vi "FGV_SQL_pinion_ID_buffer.vi"(4 "SQL_result":variant[][](array[variant]), 6 "connection reference":T2, 7 "options":T3, 8 "error_in":errorcluster, 9 "station":T1, 10 "PINION_ID":string, 11 "PINION_SERIAL":string) -> (0 "error_out":errorcluster, 2 "Pinion exists?":bool, 3 "ID_out":string)   [LabVIEW 2020]
uses:
  FGV_SQL_pinion_ID_buffer.ctl
  <vilib>/addons/database/Connection.llb/Conn ObjectReference.ctl
  STATION/station.ctl
  SQL_pinion_ID_buffer_all_info.ctl
  <vilib>/addons/database/NI_Database_API.lvlib
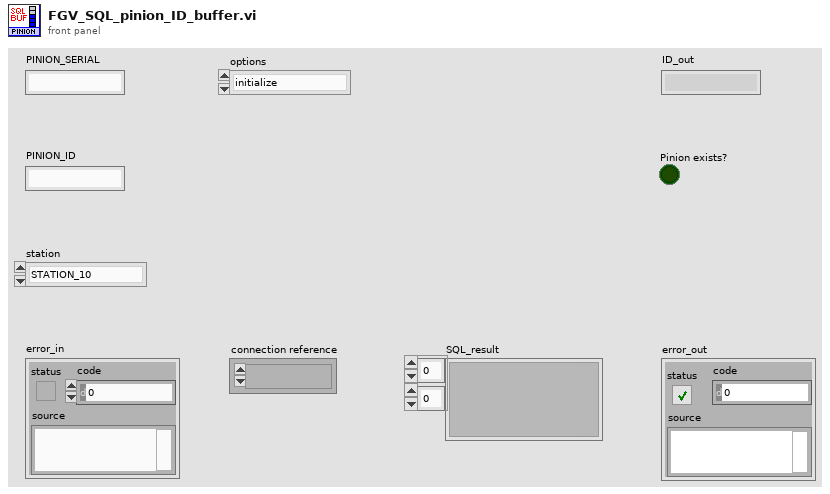
[diagram p1: front panel]
types:
  T1 = typedef "station.ctl" = enum16{"STATION_10", "STATION_20", "STATION_30", "STATION_40", "STATION_50", "STATION_60", "STATION_70", "STATION_80", "STATION_90", "STATION_100", "STATION_110", "STATION_120", "STATION_165", "MAIN"}
  T2 = typedef "NI_Database_API.lvlib/Conn ObjectReference.ctl" = refnum<k1>
  T3 = typedef "FGV_SQL_pinion_ID_buffer.ctl" = enum16{"initialize", "buffer_pinion_ID", "buffer_pinion_ID_SQL", "get_ID_for_name"}
  T4 = typedef "SQL_pinion_ID_buffer_all_info.ctl" = cluster{"PINION_SERIAL_and_ID":string[][], "PINION_SERIAL_and_ID_buffer_pos":i32, "PINION_SERIAL_and_ID_buffer_max_size":i32}
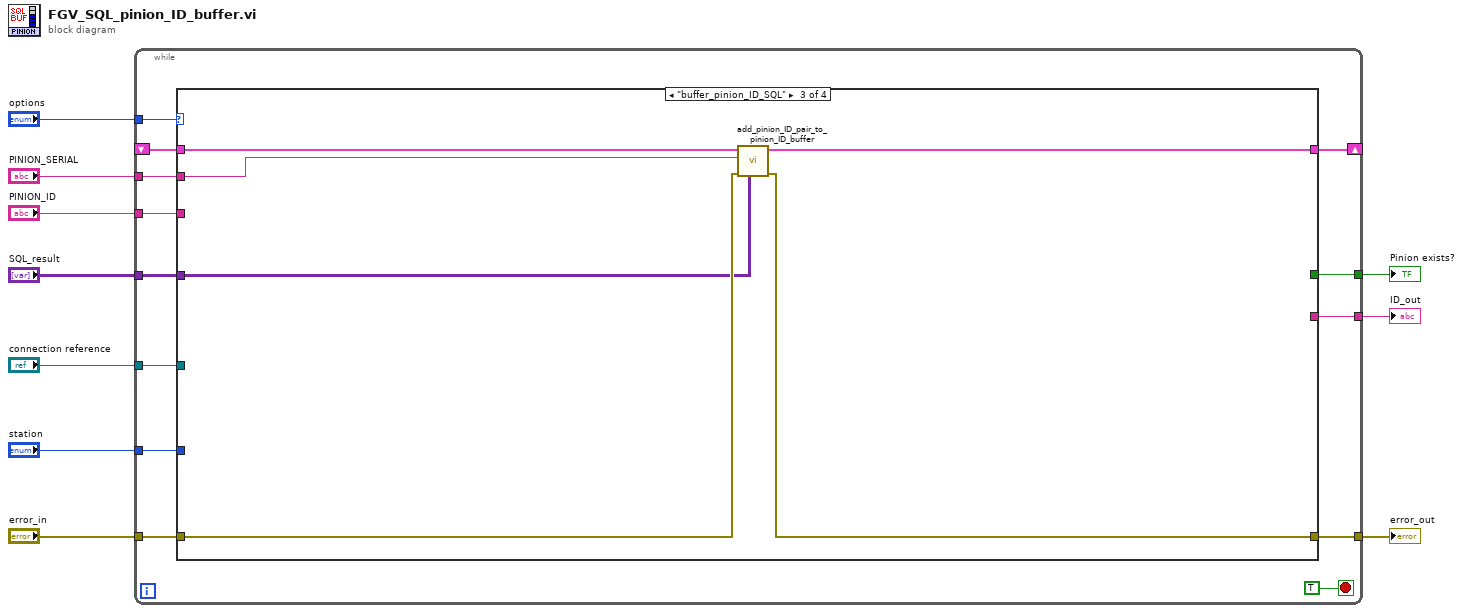
[diagram p0: block diagram]
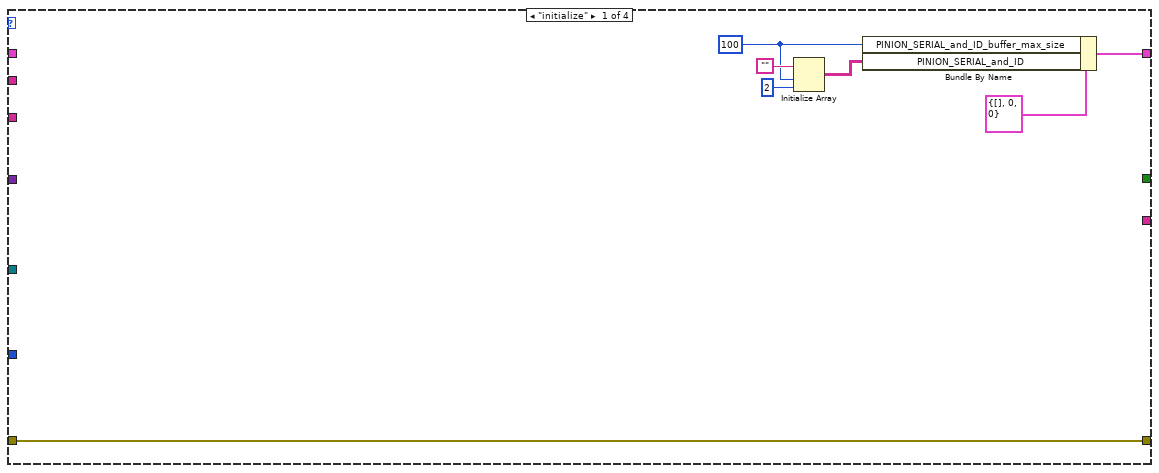
[diagram p2: hidden frame]
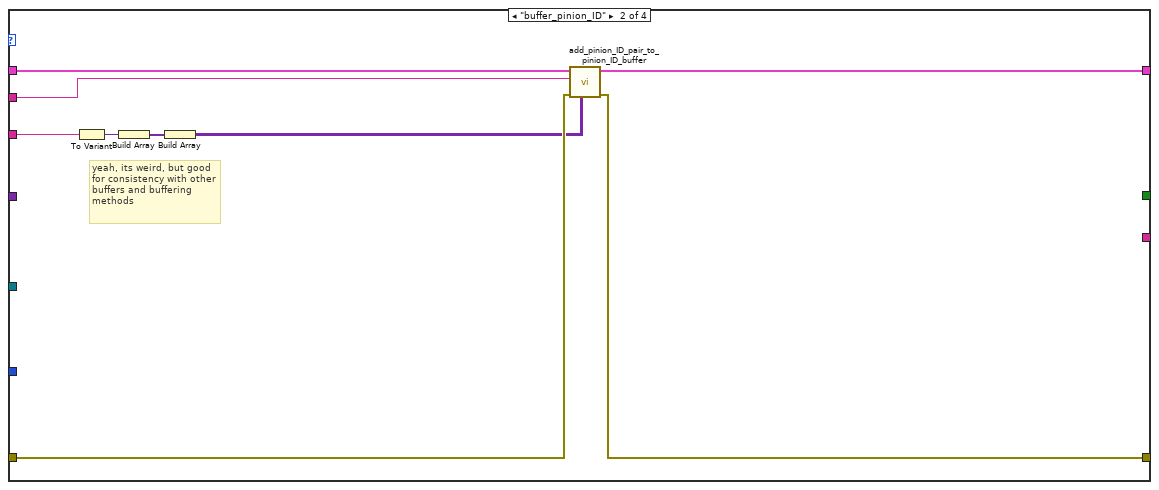
[diagram p3: hidden frame]
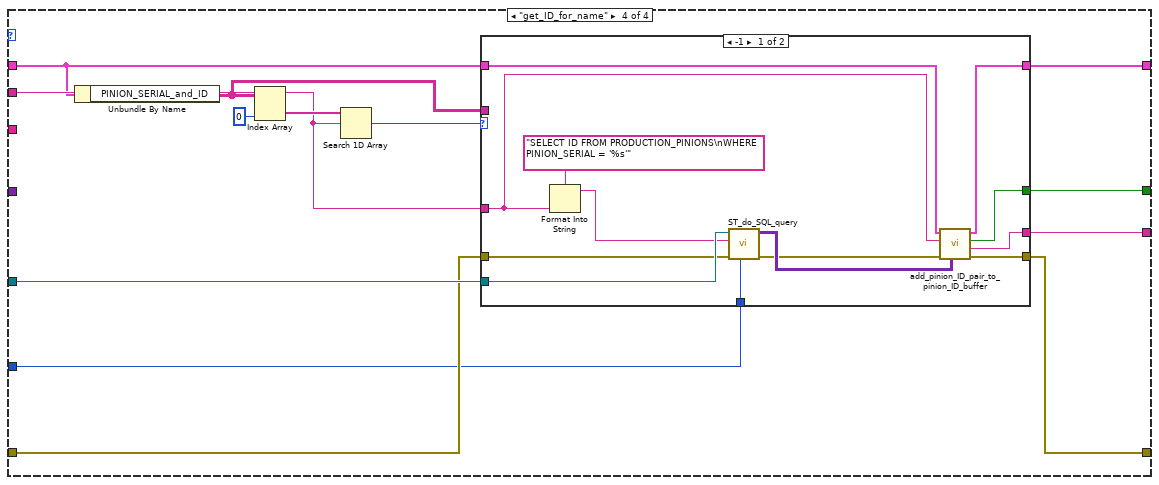
[diagram p4: hidden frame]
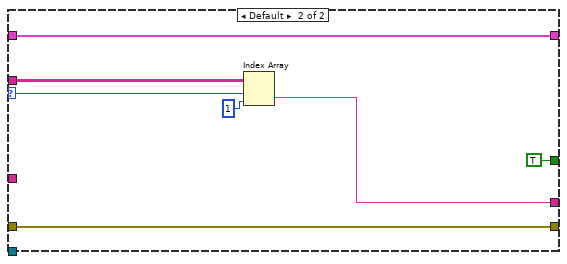
[diagram p5: hidden frame]
diagram:
  n1 = while {
    tunnel: "options" -> [w22]
    tunnel: [w21] -> w10
    tunnel: "error_in" -> [w20]
    shift-right: [w19] -> _
    shift-left: _ -> [w18]
    tunnel: "connection reference" -> [w16]
    tunnel: "PINION_SERIAL" -> [w17]
    tunnel: [w15] -> w5
    tunnel: [w14] -> w4
    tunnel: "station" -> [w13]
    tunnel: "PINION_ID" -> [w12]
    tunnel: "SQL_result" -> [w11]
    stop <- TRUE stop-if-true
    n2 = case shown="\"buffer_pinion_ID_SQL\"" w22 {
      tunnel: [w30 w36 w42 w50] -> w21
      tunnel: w20 -> [w30 w33 w41 w51]
      tunnel: [w24 w37 w43 w48] -> w19
      tunnel: w18 -> [_ w38 w44 w49]
      tunnel: w17 -> [_ w39 w45 w52]
      tunnel: w16 -> [_ _ _ w53]
      tunnel: [_ _ _ w54] -> w15
      tunnel: [_ _ _ w47] -> w14
      tunnel: w13 -> [_ _ _ w46]
      tunnel: w12 -> [_ w35 _ _]
      tunnel: w11 -> [_ _ w40 _]
      frame "initialize" {
        w26 = 100 ("dimension size")
        n3 = Initialize Array("", w26, 2 ("dimension size")) -> (w29:string[][])
        n4 = Bundle By Name(cluster=T4 {"PINION_SERIAL_and_ID"=[], "PINION_SERIAL_and_ID_buffer_pos"=0, "PINION_SERIAL_and_ID_buffer_max_size"=0} ("SQL_pinion_ID_buffer_all_info"), "PINION_SERIAL_and_ID_buffer_max_size"=w26, "PINION_SERIAL_and_ID"=w29) -> (w24:T4)
      }
      frame "buffer_pinion_ID" {
        # "yeah, its weird, but good for consistency with other buffers and buffering methods"
        n5 = To Variant(anything=w35) -> (Variant=w34:variant)
        n6 = Build Array(w34) -> (w32:variant[])
        n7 = Build Array(w32) -> (w31:variant[][])
        n8 = call "add_pinion_ID_pair_to_pinion_ID_buffer.vi"("recordset_in"=w31, "error_in"=w33, "PINION_SERIAL"=w39, "SQL_pinion_ID_buffer_all_info_in"=w38) -> ("error_out"=w36:errorcluster, "SQL_pinion_ID_buffer_all_info_out"=w37:T4)  [unwired: 4 in, 2 out]
      }
      frame "buffer_pinion_ID_SQL" {
        n9 = call "add_pinion_ID_pair_to_pinion_ID_buffer.vi"("recordset_in"=w40, "error_in"=w41, "PINION_SERIAL"=w45, "SQL_pinion_ID_buffer_all_info_in"=w44) -> ("error_out"=w42:errorcluster, "SQL_pinion_ID_buffer_all_info_out"=w43:T4)  [unwired: 4 in, 2 out]
      }
      frame "get_ID_for_name" {
        n10 = Unbundle By Name(w49) -> ("PINION_SERIAL_and_ID"=w55:string[][])
        n11 = Index Array(array=w55, index (col)=0 ("disabled index (col)")) -> (element=w57:string[])  [unwired: 1 in]
        n12 = Search 1D Array(1D array=w57, element=w52) -> (index of element=w56:i32)  [unwired: 1 in]
        n13 = case shown="-1" w56 {
          selector: w56 -> [_ w78]
          tunnel: w55 -> [_ w77]
          tunnel: [w66 w75] -> w54
          tunnel: w53 -> [w65 _]
          tunnel: w52 -> [w67 _]
          tunnel: w51 -> [w62 w74]
          tunnel: [w70 w74] -> w50
          tunnel: w49 -> [w69 w73]
          tunnel: [w68 w73] -> w48
          tunnel: [w64 TRUE ("Part exists?")] -> w47
          tunnel: w46 -> [w60 _]
          frame -1 {
            n14 = Format Into String(format string="SELECT ID FROM PRODUCTION_PINIONS\nWHERE PINION_SERIAL = '%s'", w67) -> (resulting string=w61:string)  [unwired: 2 in, 1 out]
            n15 = call "ST_do_SQL_query.vi"("station"=w60, "error_in"=w62, "SQL_query"=w61, "SQL_connection_reference"=w65) -> ("error_out"=w59:errorcluster, "recordset_out"=w63:variant[][])  [unwired: 6 in]
            n16 = call "add_pinion_ID_pair_to_pinion_ID_buffer.vi"("recordset_in"=w63, "error_in"=w59, "PINION_SERIAL"=w67, "SQL_pinion_ID_buffer_all_info_in"=w69) -> ("error_out"=w70:errorcluster, "PINION_ID_out"=w66:string, "Pinion exists?"=w64:bool, "SQL_pinion_ID_buffer_all_info_out"=w68:T4)  [unwired: 4 in]
          }
          frame Default {
            n17 = Index Array(array=w77, index (row)=w78, index (col)=1 ("disabled index (col)")) -> (element=w75:string)
          }
        }
      }
    }
  }
  "error_out" <- w10
  "ID_out" <- w5
  "Pinion exists?" <- w4
